vi "框中控件.vi"(8 "error in (no error)":errorcluster caption="错误输入（无错误）", 10 "结束坐标":cluster{"Horizontal":i32, "Vertical":i32}, 11 "程序响应 输入":refnum<class "程序响应.lvclass">) -> (0 "error out":errorcluster caption="错误输出", 3 "程序响应 输出":refnum<class "程序响应.lvclass">)   [LabVIEW 2018, in "程序响应.lvlib" / "程序响应.lvclass"]
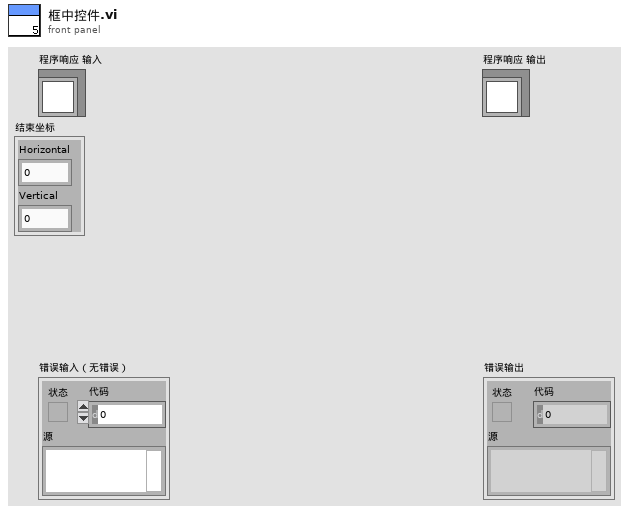
[diagram p1: front panel]
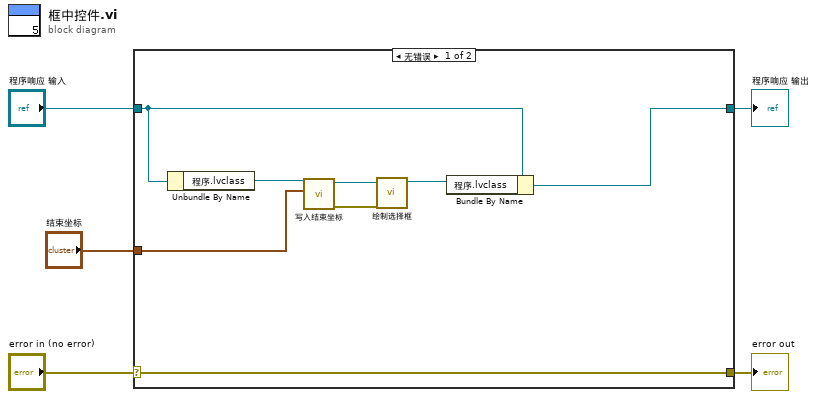
[diagram p0: block diagram]
diagram:
  n1 = case shown="无错误" "error in (no error)" {
    selector: "error in (no error)" -> [w13 w15]
    tunnel: [w13 w15] -> w4
    tunnel: [w6 w14] -> w2
    tunnel: "程序响应 输入" -> [w7 w14]
    tunnel: "结束坐标" -> [w11 _]
    frame No Error {
      n2 = Unbundle By Name(w7) -> ("程序.lvclass"=w12:refnum<class "程序.lvclass">)
      n3 = call-dynamic "写入结束坐标.vi"("结束坐标"=w11, "程序输入"=w12) -> ("error out"=w9:errorcluster, "程序输出"=w10:refnum<class "程序.lvclass">)  [unwired: 8 in]
      n4 = call-dynamic "绘制选择框.vi"("error in (no error)"=w9, "程序 输入"=w10) -> ("程序 输出"=w8:refnum<class "程序.lvclass">)  [unwired: 8 in, 1 out]
      n5 = Bundle By Name(cluster=w7, "程序.lvclass"=w8) -> (w6:refnum<class "程序响应.lvclass">)
    }
    frame Error {
    }
  }
  "error out" <- w4
  "程序响应 输出" <- w2
